vi "result save path.vi"(9 "Result OK:T":bool, 11 "model":string="D042") -> (0 "Serial No.":string, 3 "Dup Path Out":path)   [LabVIEW 2015]
panel:
  out "Year":string
  out "MOnth":string
  out "Date":string
  out "date/time string":string
  out "month":string
  out "date":string
  out "year":string
  out "appended path":path
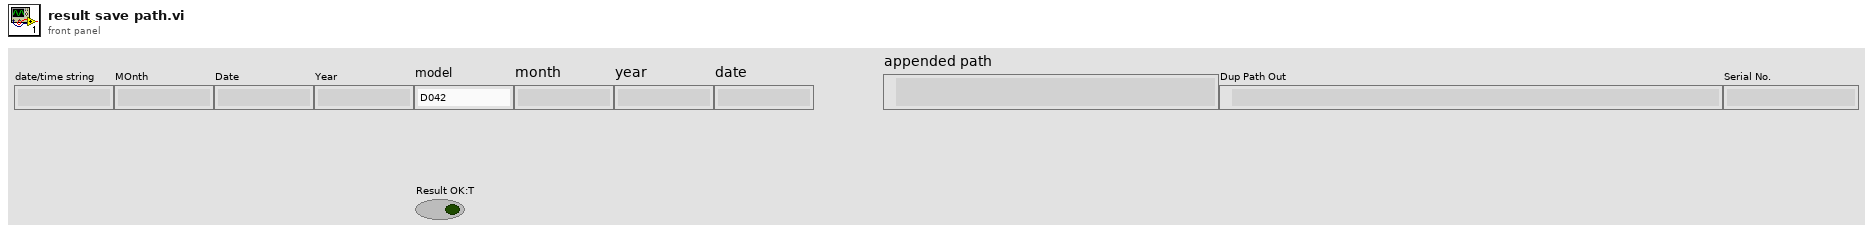
[diagram p1: front panel]
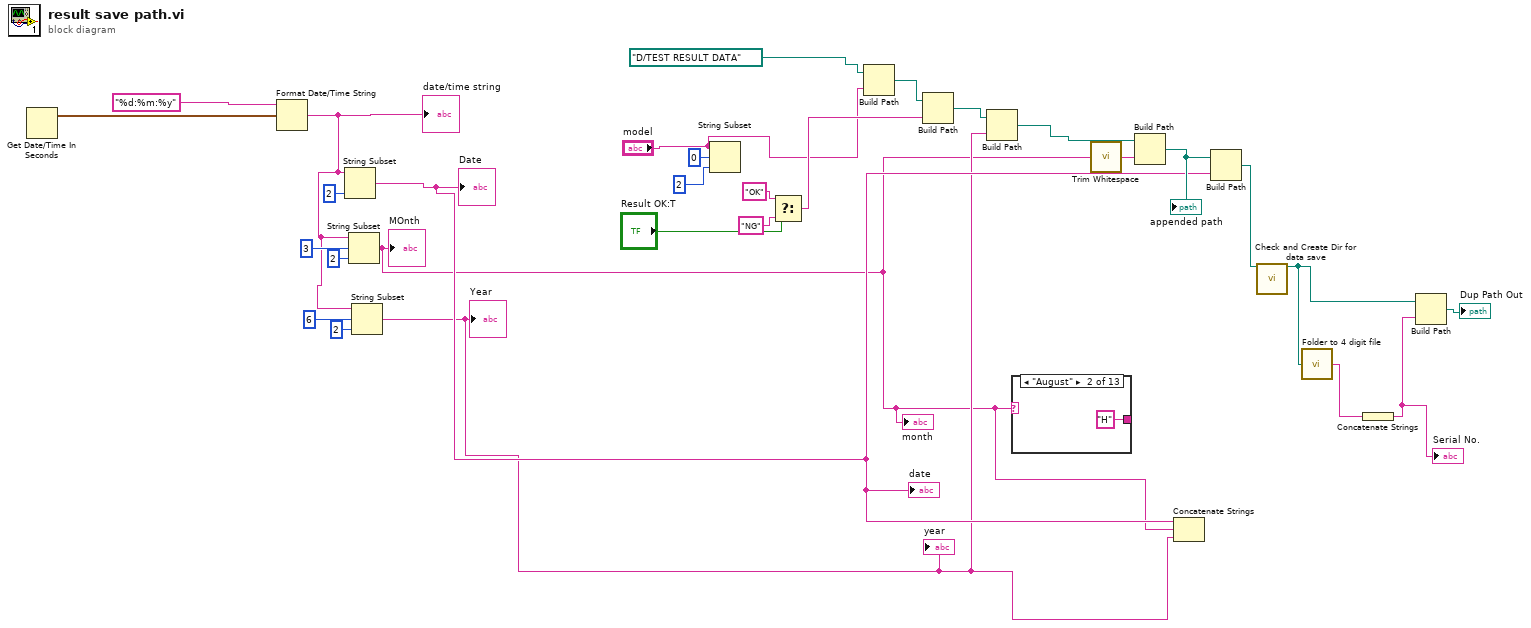
[diagram p0: block diagram]
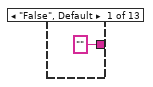
[diagram p2: hidden frame]
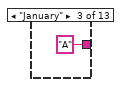
[diagram p3: hidden frame]
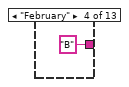
[diagram p4: hidden frame]
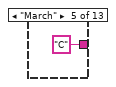
[diagram p5: hidden frame]
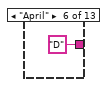
[diagram p6: hidden frame]
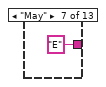
[diagram p7: hidden frame]
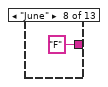
[diagram p8: hidden frame]
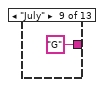
[diagram p9: hidden frame]
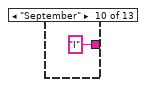
[diagram p10: hidden frame]
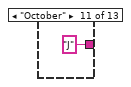
[diagram p11: hidden frame]
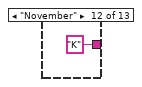
[diagram p12: hidden frame]
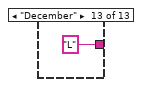
[diagram p13: hidden frame]
diagram:
  n1 = Get Date/Time In Seconds() -> (seconds since 1Jan1904=w19:timestamp)
  n2 = Format Date/Time String(time format string (%c)="%d:%m:%y", seconds (now)=w19) -> (date/time string=w12:string)  [unwired: 1 in]
  "date/time string" <- w12
  n3 = String Subset(string=w12, length (rest)=2 ("length (rest)")) -> (substring=w11:string)  [unwired: 1 in]
  "date" <- w11
  "Date" <- w11
  n4 = String Subset(string=w12, offset (0)=3, length (rest)=2 ("length (rest)")) -> (substring=w9:string)
  "month" <- w9
  "MOnth" <- w9
  n5 = String Subset(string=w12, offset (0)=6, length (rest)=2 ("length (rest)")) -> (substring=w10:string)
  "year" <- w10
  "Year" <- w10
  n6 = String Subset(string="model", offset (0)=0, length (rest)=2 ("length (rest)")) -> ()  [unwired: 1 out]
  n7 = Select(t="OK" ("Year"), s="Result OK:T", f="NG" ("Year")) -> (s? t:f=w6:string)
  n8 = Build Path(base path=path "D:/TEST RESULT DATA", name or relative path="model") -> (appended path=w7:path)
  n9 = Build Path(base path=w7, name or relative path=w6) -> (appended path=w1:path)
  n10 = Build Path(base path=w1, name or relative path=w10) -> (appended path=w20:path)
  n11 = case shown="\"August\"" w9 {
    tunnel: ["" ("string") "H" ("string") "A" ("string") "B" ("string") "C" ("string") "D" ("string") "E" ("string") "F" ("string") "G" ("string") "I" ("string") "J" ("string") "K" ("string") "L" ("string")] -> _
    frame "False", Default {
    }
    frame "August" {
    }
    frame "January" {
    }
    frame "February" {
    }
    frame "March" {
    }
    frame "April" {
    }
    frame "May" {
    }
    frame "June" {
    }
    frame "July" {
    }
    frame "September" {
    }
    frame "October" {
    }
    frame "November" {
    }
    frame "December" {
    }
  }
  n12 = call <vilib>:"Trim Whitespace.vi"("string"=w9) -> ("trimmed string"=w27:string)  [unwired: 1 in]
  n13 = Build Path(base path=w20, name or relative path=w27) -> (appended path=w29:path)
  "appended path" <- w29
  n14 = Concatenate Strings(w11, w9, w10) -> ()  [unwired: 1 out]
  n15 = Build Path(base path=w29, name or relative path=w11) -> (appended path=w28:path)
  n16 = call "Check and Create Dir for data save.vi"("Path In"=w28) -> ("Dup Path Out"=w23:path)  [unwired: 12 in, 2 out]
  n17 = call "Folder to 4 digit file.vi"("path 2"=w23) -> ("decimal integer string"=w22:string)  [unwired: 2 in]
  n18 = Concatenate Strings(w22) -> (w21:string)
  "Serial No." <- w21
  n19 = Build Path(base path=w23, name or relative path=w21) -> (appended path=→"Dup Path Out":path)
